vi "example_powershell.vi"() -> ()   [LabVIEW 2019]
uses:
  dotnet_system_exec/dotnet_system_exec.lvclass
panel:
  out "StdErr":string
  out "StdOut":string
  # "This example demonstrates Powershell.exe interations, performing a series of pings to 127.0.0.1 to illustrate the asynchronous StdOut updates. \n\nThere is a ~1sec delay between pings, so the total execution time should be about 5 seconds, but you can see the StdOut messages as they are\ngenerated, as opposed to waiting for the entire operation to complete.\n\nThis also demonstrates the StdErr output by performing an intentionally invalid Copy operation, as well as a direct \"Write-Error\" operation.\n\nThe commands are followed by an \"exit\" command, which fires the \"Process Exited\" event and stops this VI."
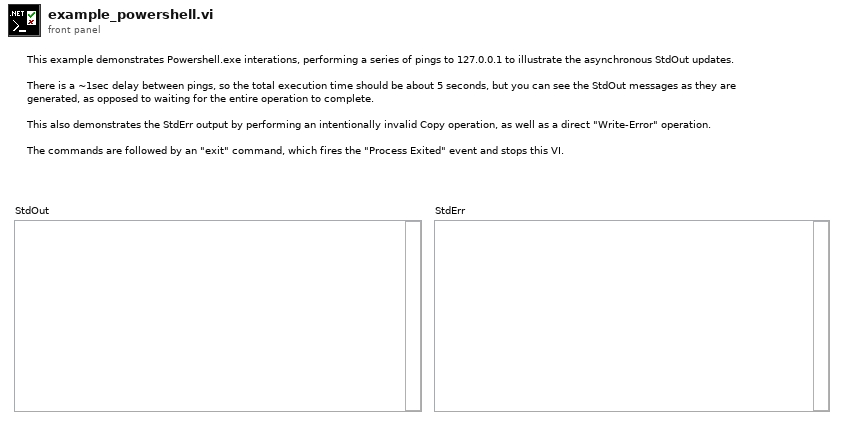
[diagram p1: front panel]
types:
  T1 = cluster{"stdout event":refnum<user-event>, "stderr event":refnum<user-event>, "ProcessExit event":refnum<user-event>}
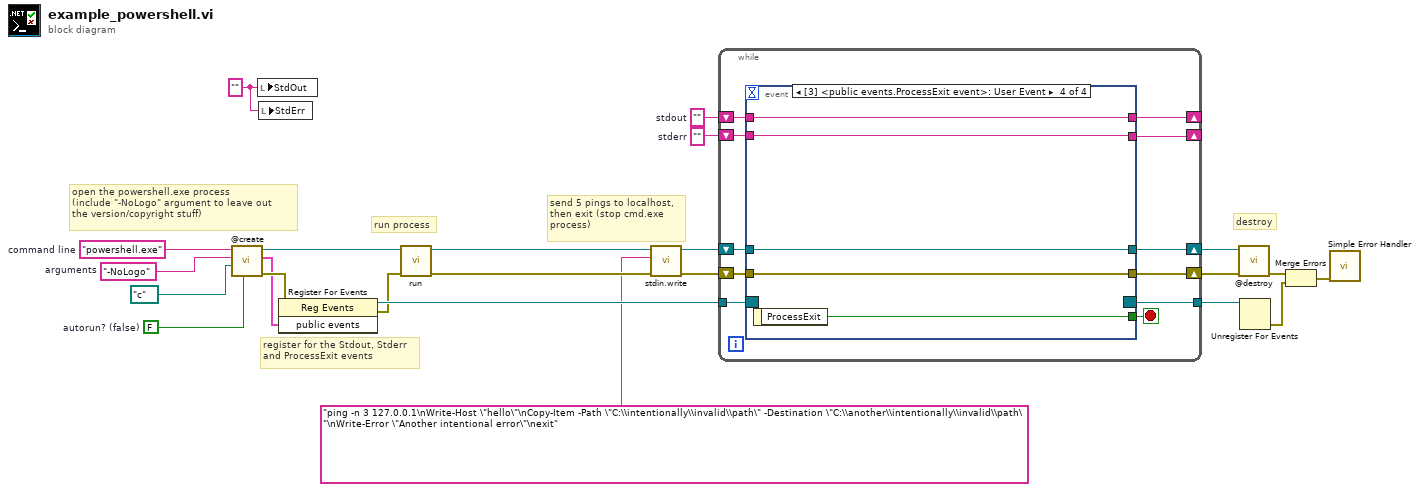
[diagram p0: block diagram]
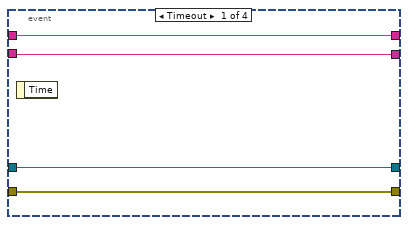
[diagram p2: hidden frame]
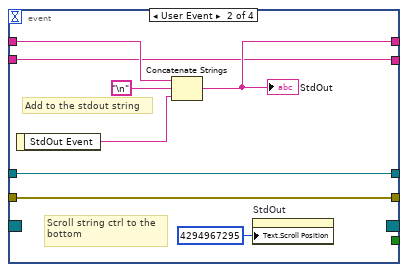
[diagram p3: hidden frame]
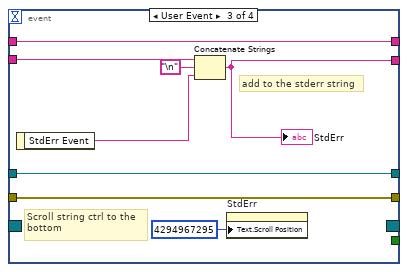
[diagram p4: hidden frame]
diagram:
  w6 = FALSE  # autorun? (false)
  w7 = "" ("Process File Name")
  w9 = ""  # stderr
  w13 = "-NoLogo"  # arguments
  w14 = ""  # stdout
  w15 = "powershell.exe"  # command line
  # "send 5 pings to localhost,\nthen exit (stop cmd.exe \nprocess)"
  # "destroy"
  # "register for the Stdout, Stderr \nand ProcessExit events"
  # "run process"
  # "open the powershell.exe process\n(include \"-NoLogo\" argument to leave out\nthe version/copyright stuff)"
  n1 = call "@create.vi"("autorun? (false)"=w6, "working directory (c:\\)"=path "c:/" ("working directory"), "arguments (\"\")"=w13, "command line (cmd.exe)"=w15) -> ("error out"=w12:errorcluster, "public events"=w10:T1, "dotnet_system_exec out"=w22:refnum<class "dotnet_system_exec.lvclass">)  [unwired: 5 in]
  n2 = local write "StdOut"(w7) -> ()
  n3 = local write "StdErr"(w7) -> ()
  n4 = register-events(error in=w12, w10) -> (reference out=w21:refnum<event-registration>, error out=w11:errorcluster)  [unwired: 1 in]
  n5 = call "run.vi"("error in (no error)"=w11, "dotnet_system_exec in"=w22) -> ("error out"=w4:errorcluster, "dotnet_system_exec out"=w5:refnum<class "dotnet_system_exec.lvclass">)  [unwired: 8 in]
  n6 = call-dynamic "stdin.write.vi"("error in (no error)"=w4, "stdin"="ping -n 3 127.0.0.1\nWrite-Host \"hello\"\nCopy-Item -Path \"C:\\intentionally\\invalid\\path\" -Destination \"C:\\another\\intentionally\\invalid\\path\"\nWrite-Error \"Another intentional error\"\nexit", "dotnet_system_exec in"=w5) -> ("error out"=w2:errorcluster, "dotnet_system_exec out"=w3:refnum<class "dotnet_system_exec.lvclass">)  [unwired: 7 in]
  n7 = while {
    shift-right: [w34] -> w23
    shift-left: w3 -> [w33]
    shift-right: [w31] -> w19
    shift-left: w2 -> [w32]
    tunnel: w21 -> [w30]
    tunnel: [w29] -> w20
    shift-right: [w27] -> _
    shift-left: w14 -> [w28]
    shift-right: [w24] -> _
    shift-left: w9 -> [w25]
    stop <- w26 stop-if-true
    n8 = event shown="[3] <public events.ProcessExit event>: User Event" {
      selector: w30 -> [_ _ _ _]
      dyn-events: [_ _ _ _] -> w29
      timeout: _ -> [_ _ _ _]
      tunnel: [w38 w46 w54 w56] -> w34
      tunnel: w33 -> [w38 w46 w54 w56]
      tunnel: w32 -> [w37 w45 w53 w55]
      tunnel: [w37 w45 w53 w55] -> w31
      tunnel: w28 -> [w36 w42 w49 w57]
      tunnel: [w36 w43 w49 w57] -> w27
      tunnel: [_ _ _ w59] -> w26
      tunnel: w25 -> [w35 w40 w50 w58]
      tunnel: [w35 w40 w48 w58] -> w24
      event Timeout {
        n9 = event-data() -> ()  [unwired: 1 in, 1 out]
      }
      event User Event {
        # "Scroll string ctrl to the \nbottom"
        # "Add to the stdout string"
        n10 = event-data() -> ("StdOut Event"=w41:string)  [unwired: 1 in]
        n11 = Concatenate Strings(w42, "\n", w41) -> (w43:string)
        "StdOut" <- w43
        n12 = property on="StdOut" class="Str"("Text.Scroll Position"=u32 4294967295) -> ()  [unwired: 2 in, 2 out]
      }
      event User Event {
        # "Scroll string ctrl to the \nbottom"
        # "add to the stderr string"
        n13 = event-data() -> ("StdErr Event"=w51:string)  [unwired: 1 in]
        n14 = Concatenate Strings(w50, "\n", w51) -> (w48:string)
        "StdErr" <- w48
        n15 = property on="StdErr" class="Str"("Text.Scroll Position"=u32 4294967295) -> ()  [unwired: 2 in, 2 out]
      }
      event User Event {
        n16 = event-data() -> ("ProcessExit"=w59:bool)  [unwired: 1 in]
      }
    }
  }
  n17 = call-dynamic "@destroy.vi"("error in (no error)"=w19, "dotnet_system_exec in"=w23) -> ("error out"=w18:errorcluster)  [unwired: 8 in, 1 out]
  n18 = Unregister For Events(event registration refnum=w20) -> (error out=w17:errorcluster)  [unwired: 1 in]
  n19 = Merge Errors(w18, w17) -> (w16:errorcluster)
  n20 = call <vilib>:"Simple Error Handler.vi"("error in (no error)"=w16) -> ()  [unwired: 4 in, 5 out]
